vi "MSEditor_SubVI_InSelections.vi"(1 "Selections":cluster{"Start":u32, "End":u32}[](array[cluster]), 2 "Numeric":u32) -> (0 "In Selection?":bool)   [LabVIEW 2016]
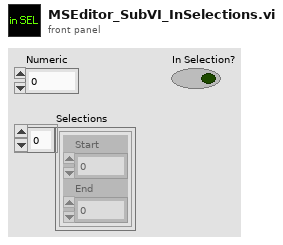
[diagram p1: front panel]
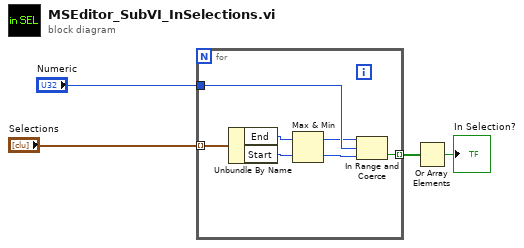
[diagram p0: block diagram]
diagram:
  n1 = for {
    tunnel: "Selections" -> [w11] mode=indexing
    tunnel: "Numeric" -> [w10]
    tunnel: [w9] -> w3 mode=indexing
    n2 = Unbundle By Name(w11) -> ("End"=w8:u32, "Start"=w7:u32)
    n3 = Max & Min(x=w8, y=w7) -> (max(x,y)=w6:u32, min(x,y)=w5:u32)
    n4 = In Range and Coerce(upper limit=w6, x=w10, lower limit=w5) -> (In Range?=w9:bool)  [unwired: 1 out]
  }
  n5 = Or Array Elements(Boolean array=w3) -> (logical OR=→"In Selection?":bool)
